vi "2ndStrikerV2.vi"(0 "command\nenum":T11, 1 "Toral de n\natacantes":i32, 2 "Total de robos":u32[](array[numeric]), 3 "N atacantes":u32[](array[numeric]), 4 "AI Parameters":T1={"GotoKick"={"Dist do cone a frente"=150.0, "attacker farback"=1500.0, "Perto"=300.0, "min dist to kick"=150.0, "kick eps"=0.0, "Time to transition"=0.05}, "Attacker"={"CC chute"=0.09, "CC passe"=0.045, "Kick Force"=100.0, "ball-robot Kick"=200.0, "ball-robot Pass"=0.3, "drible\nAttk"=FALSE}, "Defender"={"D max"=1700.0, "Vel p/ robô av"=1000.0, "Kick Force"=100.0, "D atk-def"=0.0, "D farback"=0.0, "drible\ndef"=FALSE, "drible\ngoalie"=FALSE}, "Timeout"={"Field/v in x"=6.0, "Dist Robots"=300, "Dist up in y"=300}, "Pose Striker"={"dist"=200.0, "Numeric"=-4.0, "dist 2"=200.0, "drible\nstriker"=FALSE}, "Dist Stop"=300.0, "D ball out"=200, "D central gap "=150.0, "T pass"=0.0, "Force ++"=0.0, "range kick"=0.0, "Chute alto"=TRUE, "Marcador novo"=TRUE, "drible"=FALSE, "D drible"=300.0} {"D drible" format="%#_13g"; "D central gap" format="%#_13g"; "Dist Stop" format="%#_13g"; "Pose Striker"."Numeric" format="%#_13g"; "Defender"."Kick Force" format="%#_13g"; "Defender"."Vel p/ robô av" format="%#_13g"; "Attacker"."ball-robot Kick" format="%#_13g"; "Attacker"."Kick Force" format="%#_13g"; "Attacker"."CC passe" format="%#_13g"; "Attacker"."CC chute" format="%#_13g"; "GotoKick"."kick eps" format="%#_13g"; "GotoKick"."min dist to kick" format="%#_13g"; "GotoKick"."Perto" format="%#_13g"; "GotoKick"."attacker farback" format="%#_13g"; "GotoKick"."Dist do cone a frente" format="%#_13g"}, 5 "Robot":T2={"id"=0, "function"=enum."Attacker", "x"=0.0, "y"=0.0, "orientation"=0.0, "v_tangent"=0.0, "v_normal"=0.0, "v_ang"=0.0, "kick_x"=0.0, "kick_z"=0.0, "dribble"=FALSE, "Timestamp"=timestamp(0 s since 1904-01-01), "estimatives"={"est_v_tangent"=0.0, "est_v_normal"=0.0, "est_vx"=0.0, "est_vy"=0.0, "Pos Robot Est"=[]}, "dest_x_kick"=0.0, "dest_y_kick"=0.0, "Gap Coord"=[], "States"=enum."GoToTangent", "Path "=[], "Path  Smooth"=[], "Dest"=[]}, 7 "Field defense":dbl[](array[numeric]), 9 "IA Input":T7={"our_robots"=[], "enemy_robots"=[], "balls"=[], "geometry"={"line_width"=0, "field_length"=0, "field_width"=0, "boundary_width"=0, "referee_width"=0, "goal_width"=0, "goal_depth"=0, "goal_wall_width"=0, "center_circle_radius"=0, "defense_radius"=0, "defense_stretch"=0, "free_kick_from_defense_dist"=0, "penalty_spot_from_field_line_dist"=0, "penalty_line_from_spot_dist"=0}, "IA Judge"={"stage"="", "command"="", "our_goalie_id"=0.0, "enemy_goalie_id"=0.0, "command enum"=enum."Halt", "Time"=enum."Azul"}, "Received Timestamp"=timestamp(0 s since 1904-01-01), "Events"={"Touch"=FALSE, "Ball out"=FALSE, "id touch"=0.0, "Ball out of \nVision"=FALSE, "Ball inside \nGoalie area"=FALSE, "Robot not responding"=FALSE, "Robots responding status"=[1.0, 1.0, 1.0, 1.0, 1.0, 1.0], "Enemy Ball \nPossession"=FALSE, "Pass State"=FALSE, "id end of pass"=0.0, "Kick"=FALSE, "Id ini Possession"=0.0, "Ball Possesion"=FALSE, "Id Possesion"=0.0, "Direct Kick"=FALSE}}, 11 "atacando ao contrário?":bool=TRUE, 13 "geometry":T9, 14 "balls":T8[](array[typedef])) -> (6 "Robot out":T2={"id"=0, "function"=enum."Attacker", "x"=0.0, "y"=0.0, "orientation"=0.0, "v_tangent"=0.0, "v_normal"=0.0, "v_ang"=0.0, "kick_x"=0.0, "kick_z"=0.0, "dribble"=FALSE, "Timestamp"=timestamp(0 s since 1904-01-01), "estimatives"={"est_v_tangent"=0.0, "est_v_normal"=0.0, "est_vx"=0.0, "est_vy"=0.0, "Pos Robot Est"=[]}, "dest_x_kick"=0.0, "dest_y_kick"=0.0, "Gap Coord"=[], "States"=enum."GoToTangent", "Path "=[], "Path  Smooth"=[], "Dest"=[]})   [LabVIEW 2017]
uses:
  Core/AI Robot.ctl
  Functions Enum.ctl
  AttackerStates.ctl
  Path Planning/RRT/PathDests.ctl
  Path Planning/RRT/PathDest.ctl
  Command Enum.ctl
  Core/Field Size.ctl
  Core/AI Ball.ctl
  Core/AI Input.ctl
  Core/AI Judge.ctl
  Util/Events/Events.ctl
  AI Parameters.ctl
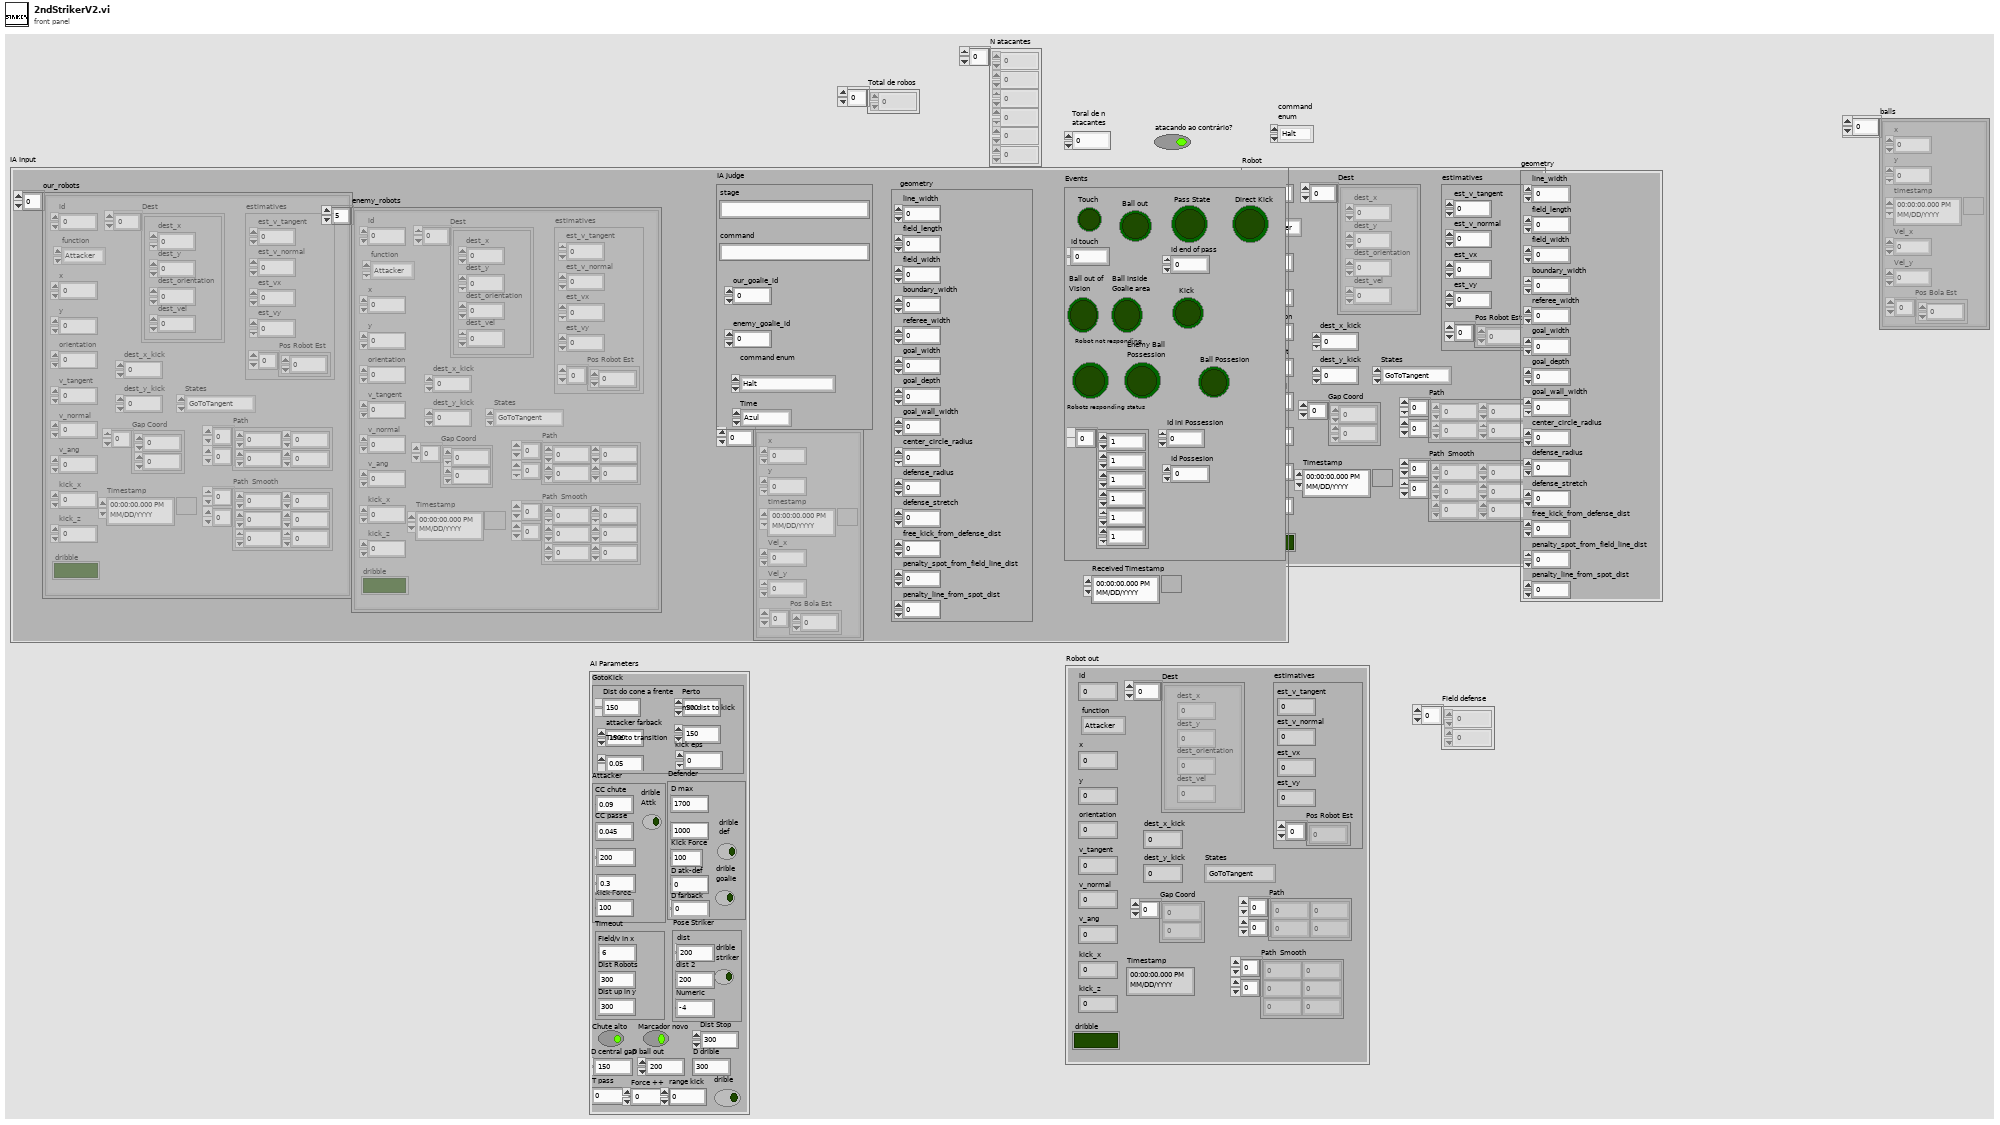
[diagram p1: front panel]
types:
  T1 = typedef "AI Parameters.ctl" = cluster{"GotoKick":cluster{"Dist do cone a frente":dbl, "attacker farback":dbl, "Perto":dbl, "min dist to kick":dbl, "kick eps":dbl, "Time to transition":dbl}, "Attacker":cluster{"CC chute":dbl, "CC passe":dbl, "Kick Force":dbl, "ball-robot Kick":dbl, "ball-robot Pass":dbl, "drible\nAttk":bool}, "Defender":cluster{"D max":dbl, "Vel p/ robô av":dbl, "Kick Force":dbl, "D atk-def":dbl, "D farback":dbl, "drible\ndef":bool, "drible\ngoalie":bool}, "Timeout":cluster{"Field/v in x":dbl, "Dist Robots":u32, "Dist up in y":u32}, "Pose Striker":cluster{"dist":dbl, "Numeric":dbl, "dist 2":dbl, "drible\nstriker":bool}, "Dist Stop":dbl, "D ball out":i32, "D central gap ":dbl, "T pass":dbl, "Force ++":dbl, "range kick":dbl, "Chute alto":bool, "Marcador novo":bool, "drible":bool, "D drible":dbl}
  T2 = typedef "AI Robot.ctl" = cluster{"id":u32, "function":T3, "x":dbl, "y":dbl, "orientation":dbl, "v_tangent":dbl, "v_normal":dbl, "v_ang":dbl, "kick_x":dbl, "kick_z":dbl, "dribble":bool, "Timestamp":timestamp, "estimatives":cluster{"est_v_tangent":dbl, "est_v_normal":dbl, "est_vx":dbl, "est_vy":dbl, "Pos Robot Est":dbl[]}, "dest_x_kick":dbl, "dest_y_kick":dbl, "Gap Coord":dbl[], "States":T4, "Path ":dbl[][], "Path  Smooth":dbl[][], "Dest":T5}
  T3 = typedef "Functions Enum.ctl" = enum16{"Attacker", "Goalie", "Defender", "Striker", "Goto 0", "Dummy", "Kicker", "ZigZag 0", "ZigZag 1", "ZigZag 2", "ZigZag 3", "ZigZag 4", "ZigZag 5", "ZigZag 6", "ZigZag 7", "ZigZag 8", ""}
  T4 = typedef "AttackerStates.ctl" = enum16{"Pass", "GoToTangent", "BallGetting", "GoToKick", ""}
  T5 = typedef "PathDests.ctl" = T6[]
  T6 = typedef "PathDest.ctl" = cluster{"dest_x":dbl, "dest_y":dbl, "dest_orientation":dbl, "dest_vel":dbl}
  T7 = typedef "AI Input.ctl" = cluster{"our_robots":T2[], "enemy_robots":T2[], "balls":T8[], "geometry":T9, "IA Judge":T10, "Received Timestamp":timestamp, "Events":T12}
  T8 = typedef "AI Ball.ctl" = cluster{"x":dbl, "y":dbl, "timestamp":timestamp, "Vel_x":dbl, "Vel_y":dbl, "Pos Bola Est":dbl[]}
  T9 = typedef "Field Size.ctl" = cluster{"line_width":u32, "field_length":u32, "field_width":u32, "boundary_width":u32, "referee_width":u32, "goal_width":u32, "goal_depth":u32, "goal_wall_width":u32, "center_circle_radius":u32, "defense_radius":u32, "defense_stretch":u32, "free_kick_from_defense_dist":u32, "penalty_spot_from_field_line_dist":u32, "penalty_line_from_spot_dist":u32}
  T10 = typedef "AI Judge.ctl" = cluster{"stage":string, "command":string, "our_goalie_id":dbl, "enemy_goalie_id":dbl, "command enum":T11, "Time":enum16{"Azul", "Amarelo"}}
  T11 = typedef "Command Enum.ctl" = enum16{"Halt", "Stop", "Force Start", "PKA Normal Start", "Prepare Kickoff Ally", "PKE Normal Start", "Prepare Kickoff Enemy", "Prepare Penalty Ally", "PPA Normal Start", "Prepare Penalty Enemy", "PPE Normal Start", "Direct Free Enemy", "Direct Free Ally", "Indirect Free Enemy", "Indirect Free Ally", "Timeout Enemy", "Timeout Ally", "Goal Enemy", "Goal Ally", "Ball Placement Enemy", "Ball Placement Ally", "Normal Half Time", "Extra Time Break", "Extra Half Time", "None", "Post Game"}
  T12 = typedef "Events.ctl" = cluster{"Touch":bool, "Ball out":bool, "id touch":dbl, "Ball out of \nVision":bool, "Ball inside \nGoalie area":bool, "Robot not responding":bool, "Robots responding status":dbl[], "Enemy Ball \nPossession":bool, "Pass State":bool, "id end of pass":dbl, "Kick":bool, "Id ini Possession":dbl, "Ball Possesion":bool, "Id Possesion":dbl, "Direct Kick":bool}
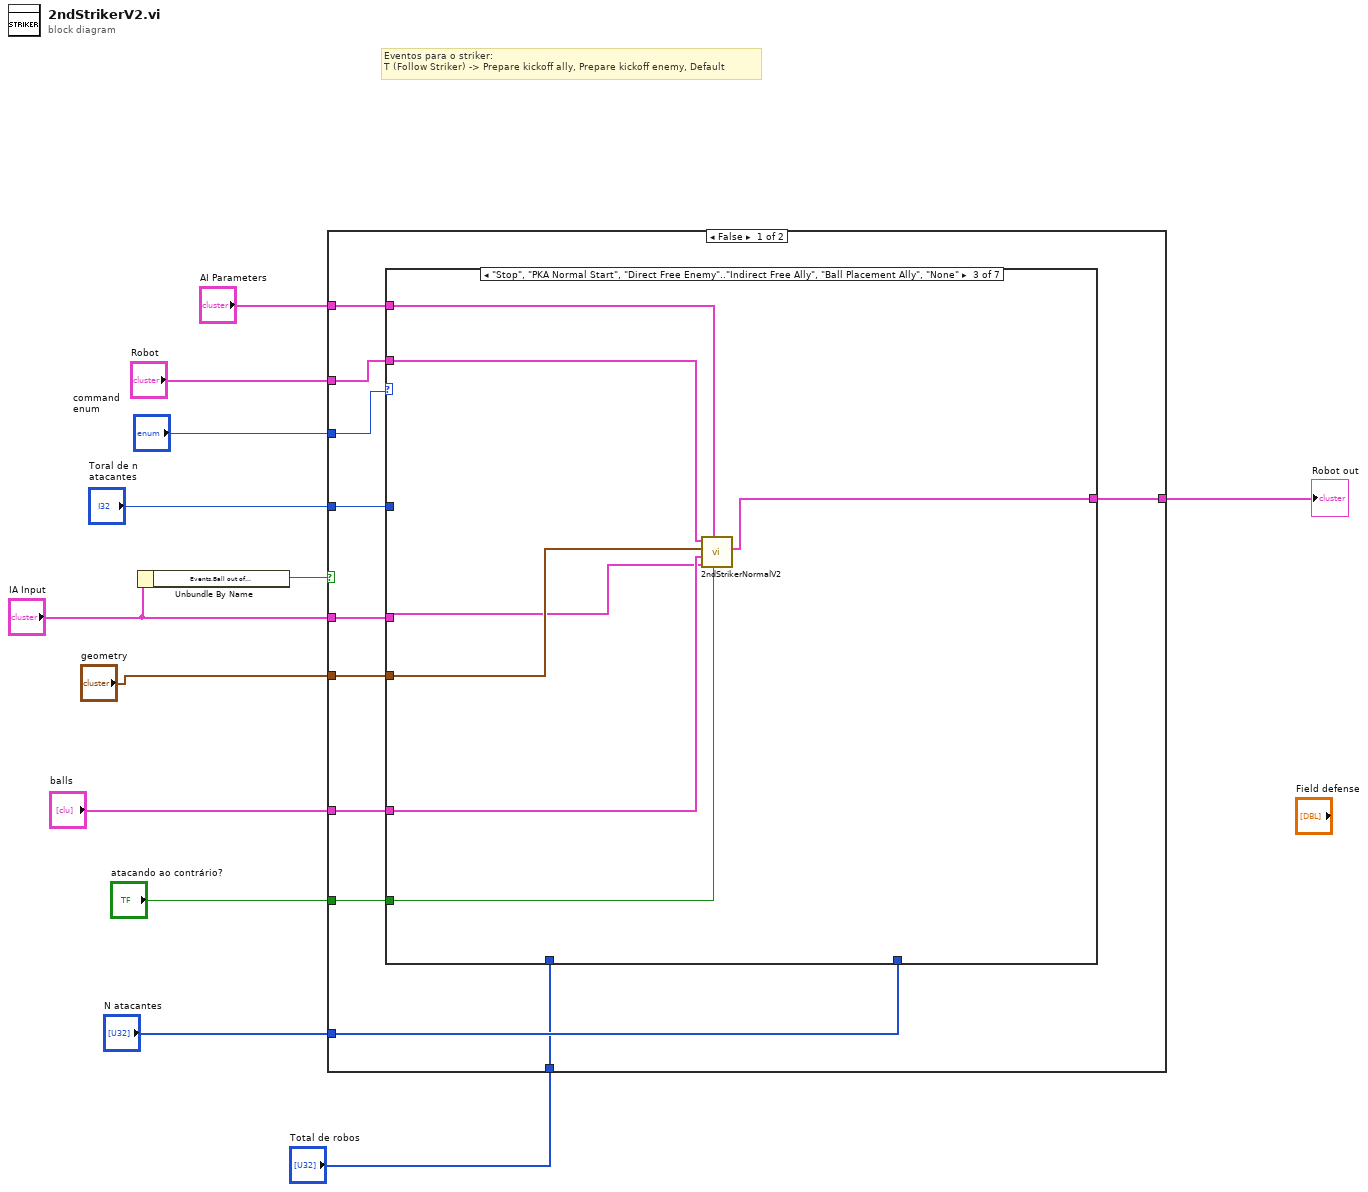
[diagram p0: block diagram]
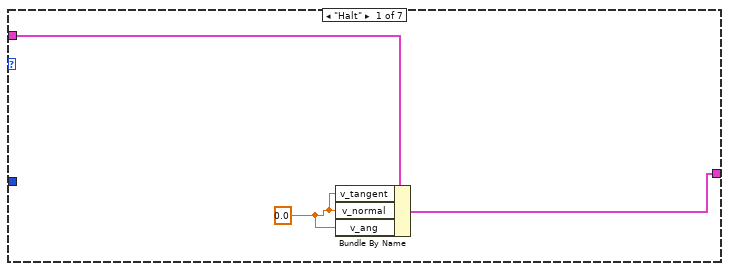
[diagram p2: hidden frame]
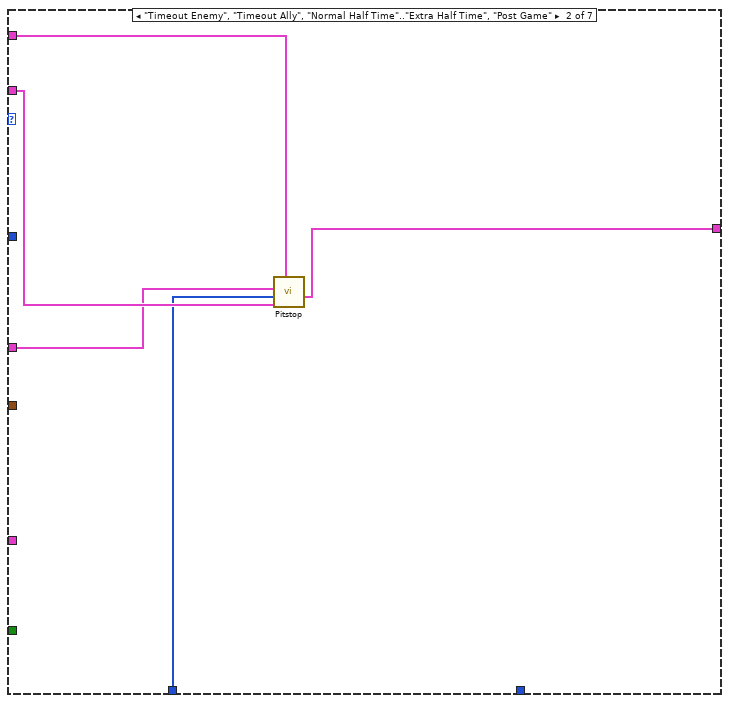
[diagram p3: hidden frame]
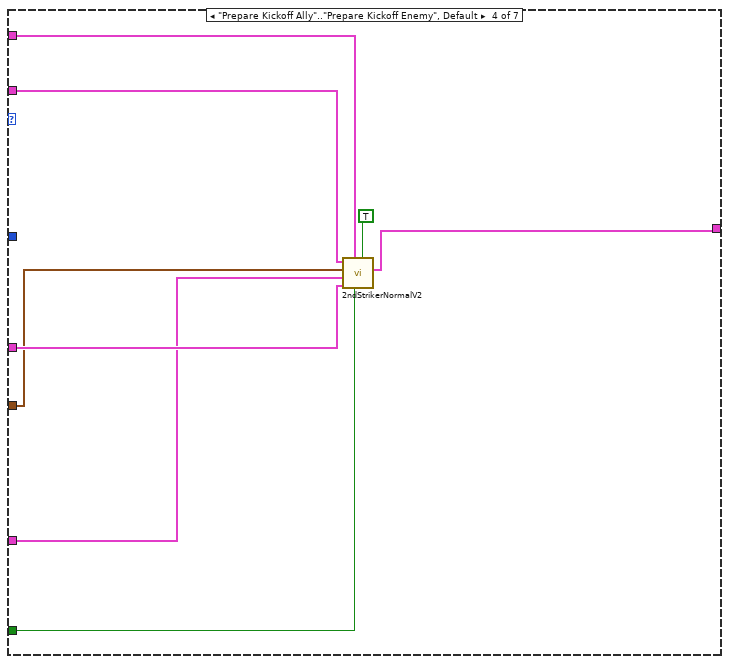
[diagram p4: hidden frame]
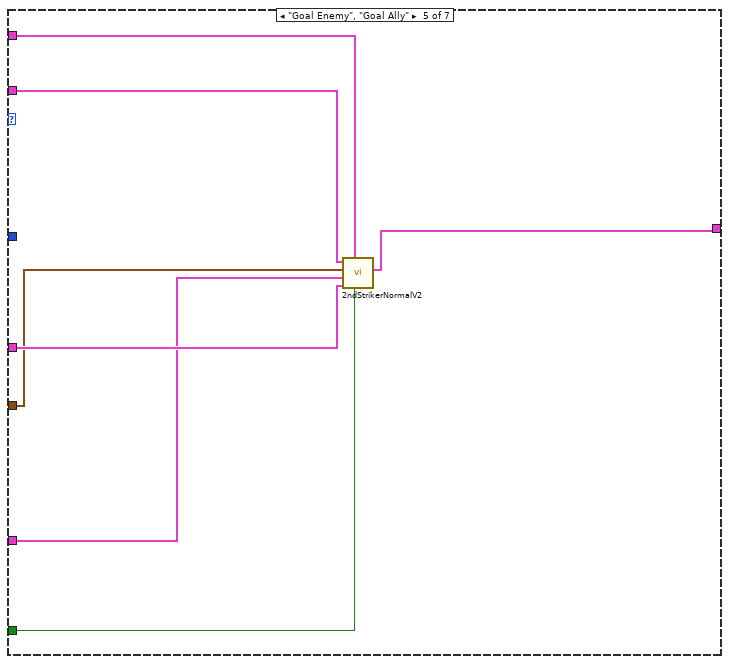
[diagram p5: hidden frame]
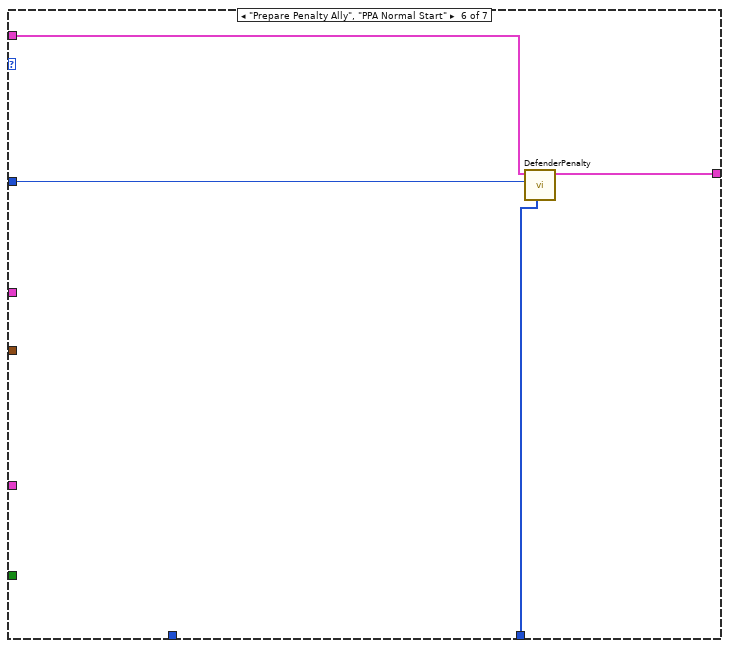
[diagram p6: hidden frame]
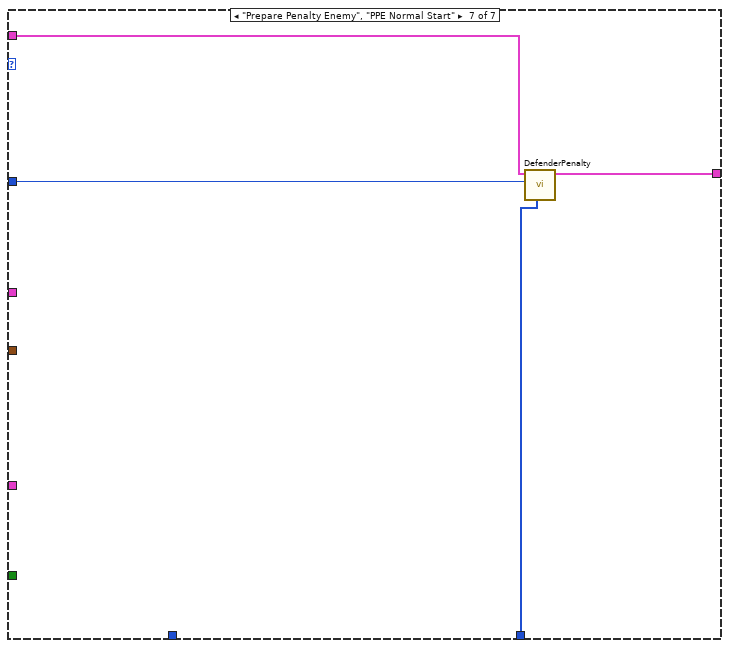
[diagram p7: hidden frame]
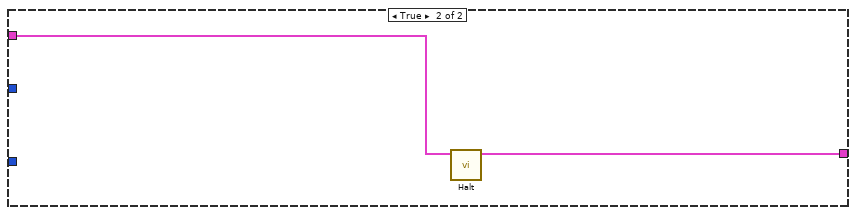
[diagram p8: hidden frame]
diagram:
  # "Eventos para o striker:\nT (Follow Striker) -> Prepare kickoff ally, Prepare kickoff enemy, Default"
  n1 = Unbundle By Name("IA Input") -> ("Events.Ball out of \nVision"=w3:bool)
  n2 = case shown="False" w3 {
    tunnel: "command\nenum" -> [w23 _]
    tunnel: "Robot" -> [w22 w62]
    tunnel: [w21 w63] -> w10
    tunnel: "geometry" -> [w20 _]
    tunnel: "balls" -> [w19 _]
    tunnel: "IA Input" -> [w18 _]
    tunnel: "atacando ao contrário?" -> [w17 _]
    tunnel: "Toral de n\natacantes" -> [w16 _]
    tunnel: "N atacantes" -> [w15 _]
    tunnel: "Total de robos" -> [w14 _]
    tunnel: "AI Parameters" -> [w13 _]
    frame False {
      n3 = case shown="\"Stop\", \"PKA Normal Start\", \"Direct Free Enemy\"..\"Indirect Free Ally\", \"Ball Placement Ally\", \"None\"" w23 {
        tunnel: w22 -> [w25 w31 w35 w41 w48 w56 w60]
        tunnel: [w24 w28 w38 w46 w53 w57 w61] -> w21
        tunnel: w20 -> [_ _ w36 w42 w49 _ _]
        tunnel: w19 -> [_ _ w37 w43 w50 _ _]
        tunnel: w18 -> [_ w29 w34 w44 w51 _ _]
        tunnel: w17 -> [_ _ w33 w45 w52 _ _]
        tunnel: w16 -> [_ _ _ _ _ w55 w59]
        tunnel: w15 -> [_ _ _ _ _ w54 w58]
        tunnel: w14 -> [_ w30 _ _ _ _ _]
        tunnel: w13 -> [_ w27 w32 w40 w47 _ _]
        frame "Halt" {
          w26 = 0.0
          n4 = Bundle By Name(cluster=w25, "v_tangent"=w26, "v_normal"=w26, "v_ang"=w26) -> (w24:T2)
        }
        frame "Timeout Enemy", "Timeout Ally", "Normal Half Time".."Extra Half Time", "Post Game" {
          n5 = call "Pitstop.vi"("AI Parameters"=w27, "Robot in"=w31, "robos"=w30, "IA State Input"=w29) -> ("Robot out"=w28:T2)  [unwired: 7 in]
        }
        frame "Stop", "PKA Normal Start", "Direct Free Enemy".."Indirect Free Ally", "Ball Placement Ally", "None" {
          n6 = call "2ndStrikerNormalV2.vi"("atacando ao contrário?"=w33, "AI Parameters"=w32, "IA Input"=w34, "balls"=w37, "Field Size in"=w36, "Robot in"=w35) -> ("Robot out"=w38:T2)  [unwired: 5 in]
        }
        frame "Prepare Kickoff Ally".."Prepare Kickoff Enemy", Default {
          n7 = call "2ndStrikerNormalV2.vi"("Stop"=TRUE, "atacando ao contrário?"=w45, "AI Parameters"=w40, "IA Input"=w44, "balls"=w43, "Field Size in"=w42, "Robot in"=w41) -> ("Robot out"=w46:T2)  [unwired: 4 in]
        }
        frame "Goal Enemy", "Goal Ally" {
          n8 = call "2ndStrikerNormalV2.vi"("atacando ao contrário?"=w52, "AI Parameters"=w47, "IA Input"=w51, "balls"=w50, "Field Size in"=w49, "Robot in"=w48) -> ("Robot out"=w53:T2)  [unwired: 5 in]
        }
        frame "Prepare Penalty Ally", "PPA Normal Start" {
          n9 = call "DefenderPenalty.vi"("N atacantes"=w54, "Total de n \natacantes"=w55, "Robot in"=w56) -> ("Robot out"=w57:T2)  [unwired: 8 in]
        }
        frame "Prepare Penalty Enemy", "PPE Normal Start" {
          n10 = call "DefenderPenalty.vi"("N atacantes"=w58, "Total de n \natacantes"=w59, "Robot in"=w60) -> ("Robot out"=w61:T2)  [unwired: 8 in]
        }
      }
    }
    frame True {
      n11 = call "Halt.vi"("Robot in"=w62) -> ("Robot out"=w63:T2)  [unwired: 10 in]
    }
  }
  "Robot out" <- w10
